vi "LMData_initialize.vi"(0 "LMData in":refnum<class "LMData.lvclass">, 1 "VISA resource name":refnum<visa-resource-name>, 2 "Labels":string[](array[string]), 3 "FileFormat":string[](array[string]), 5 "RunIdentifier":string, 7 "InstName":string, 9 "base path":path, 11 "error in (no error)":errorcluster, 12 "LevelCalibration (R0, R1, L0, L1)":dbl[](array[numeric]), 13 "Active?":bool) -> (4 "LMData out":refnum<class "LMData.lvclass">, 15 "error out":errorcluster)   [LabVIEW 2020, in "LMData.lvclass"]
uses:
  LMData.lvclass
  LMData.lvclass/LMData.ctl
  <instrlib>/Agilent 34401/Agilent 34401.lvlib
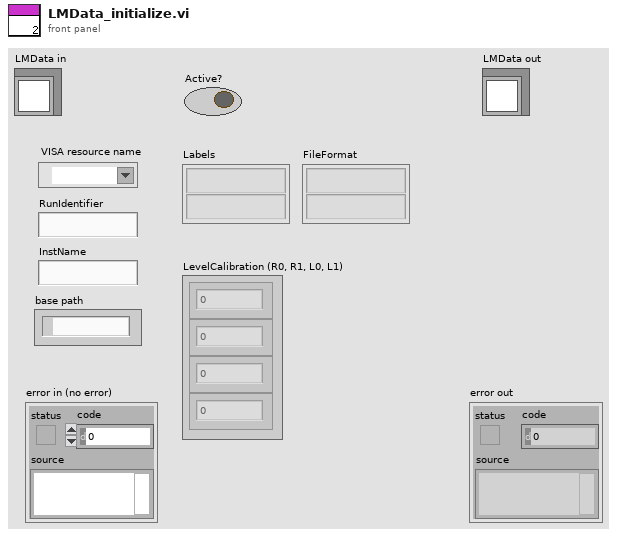
[diagram p1: front panel]
types:
  T1 = enum16{"open", "replace", "create", "open or create", "replace or create", "replace or create with confirmation"}
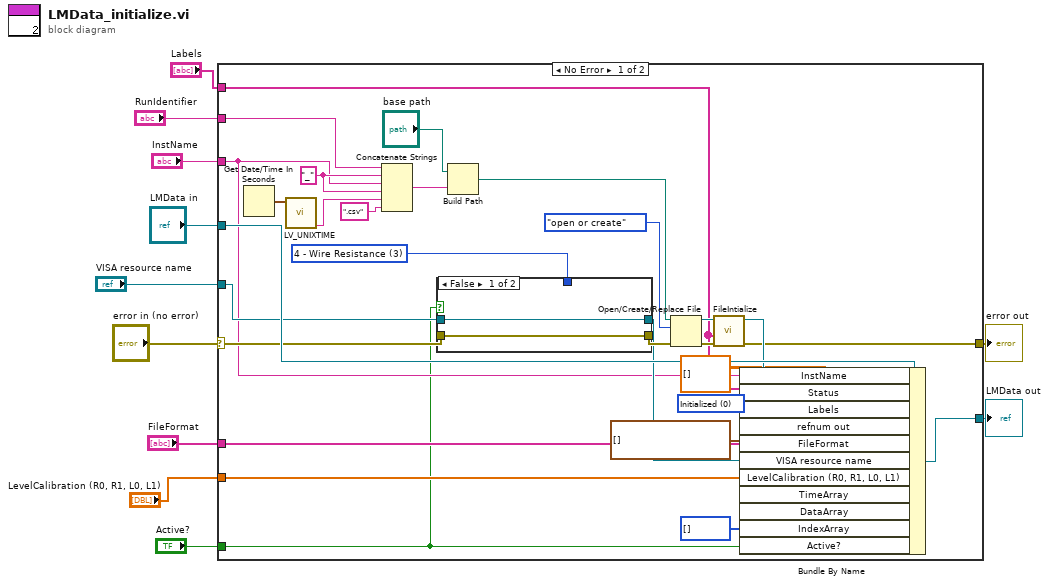
[diagram p0: block diagram]
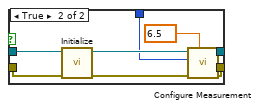
[diagram p2: hidden frame]
diagram:
  n1 = case shown="No Error" "error in (no error)" {
    selector: "error in (no error)" -> [w26 w52]
    tunnel: [w19 w52] -> w10
    tunnel: [w39 w51] -> w8
    tunnel: "LMData in" -> [w40 w51]
    tunnel: "RunIdentifier" -> [w35 _]
    tunnel: "InstName" -> [w17 _]
    tunnel: "Labels" -> [w18 _]
    tunnel: "VISA resource name" -> [w25 _]
    tunnel: "FileFormat" -> [w21 _]
    tunnel: "LevelCalibration (R0, R1, L0, L1)" -> [w13 _]
    tunnel: "Active?" -> [w12 _]
    frame No Error {
      w23 = u16 3 items=["DC Voltage", "AC Voltage", "2 - Wire Resistance", "4 - Wire Resistance", "DC Current", "AC Current", "Frequency", "Period", "Continuity", "Diode Checking", "VDC:VDC Ratio", "Temperature", "Capacitance"] ("Function (0: DC Voltage)")
      w34 = "_" ("string")
      w38 = u16 0 items=["Initialized", "Waiting", "Measuring", "Terminated"] ("Status")
      n2 = Get Date/Time In Seconds() -> (seconds since 1Jan1904=w37:timestamp)
      n3 = call "LV_UNIXTIME.vi"("current time"=w37) -> ("date/time string"=w33:string)  [unwired: 9 in, 1 out]
      n4 = Concatenate Strings(w35, w34, w17, w34, w33, ".csv" ("string")) -> (w31:string)
      n5 = case shown="False" w12 {
        tunnel: w26 -> [w41 w50]
        tunnel: w25 -> [w42 w49]
        tunnel: [w41 w46] -> w24
        tunnel: w23 -> [_ w45]
        tunnel: [w42 w43] -> w22
        frame False {
        }
        frame True {
          w44 = 6.5 items=["4.5"=4.5, "5.5"=5.5, "6.5"=6.5] ("Manual Resolution (5.5 Digits)")
          n6 = call <instrlib>:"Initialize.vi"("error in (no error)"=w50, "VISA resource name"=w49) -> ("error out"=w47:errorcluster, "VISA resource name out"=w48:refnum<visa-resource-name>)  [unwired: 8 in]
          n7 = call <instrlib>:"Configure Measurement.vi"("Manual Resolution (5.5 Digits)"=w44, "error in (no error)"=w47, "Function (0: DC Voltage)"=w45, "VISA resource name"=w48) -> ("error out"=w46:errorcluster, "VISA resource name out"=w43:refnum<visa-resource-name>)  [unwired: 6 in]
        }
      }
      n8 = Build Path(base path="base path", name or relative path=w31) -> (appended path=w30:path)
      n9 = Open/Create/Replace File(file path (use dialog)=w30, error in=w24, operation (0:open)=T1."open or create") -> (refnum out=w29:refnum<file>, error out=w28:errorcluster)  [unwired: 3 in, 1 out]
      n10 = call "FileIntialize.vi"("Error In"=w28, "Labels"=w18, "refnum in"=w29) -> ("Error Out"=w19:errorcluster, "File Refnum"=w20:refnum<file>)  [unwired: 7 in]
      n11 = Bundle By Name(cluster=w40, "InstName"=w17, "Status"=w38, "Labels"=w18, "refnum out"=w20, "FileFormat"=w21, "VISA resource name"=w22, "LevelCalibration (R0, R1, L0, L1)"=w13, "TimeArray"=timestamp[] [], "DataArray"=dbl[][] [], "IndexArray"=i64[] [], "Active?"=w12) -> (w39:refnum<class "LMData.lvclass">)
    }
    frame Error {
    }
  }
  "error out" <- w10
  "LMData out" <- w8
